vi "Mem_Release.vi"(8 "error in (no error)":errorcluster, 11 "AddrQueueIn":refnum<queue>) -> (0 "error out":errorcluster)   [LabVIEW 2019, in "Memory Data Access.lvlib"]
uses:
  Memory Data Access.lvlib
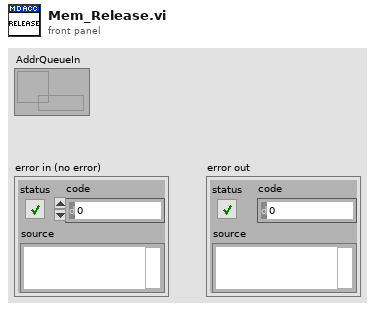
[diagram p1: front panel]
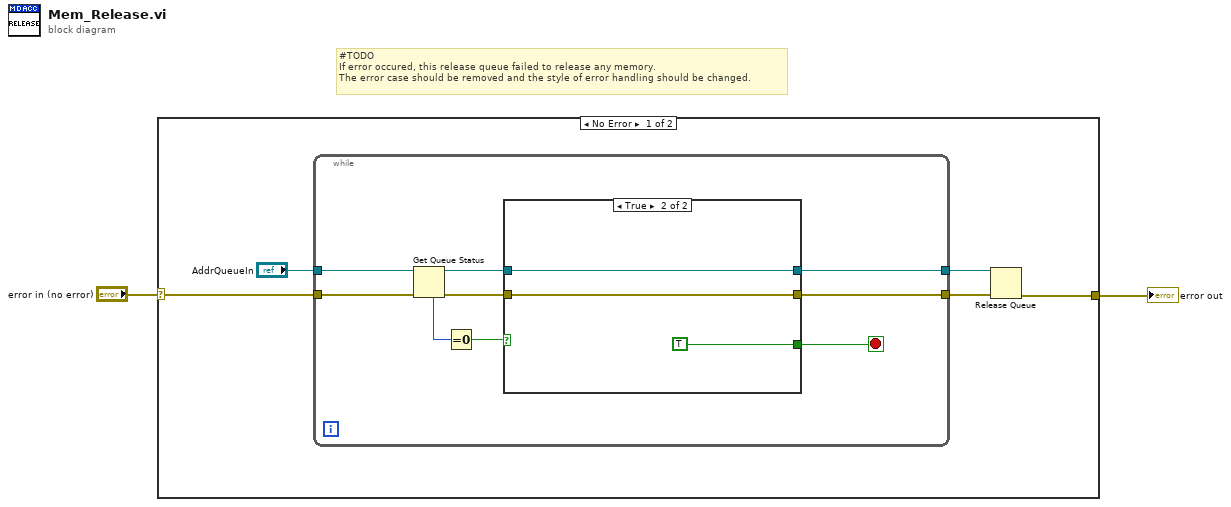
[diagram p0: block diagram]
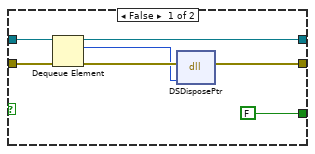
[diagram p2: hidden frame]
diagram:
  # "#TODO\nIf error occured, this release queue failed to release any memory.\nThe error case should be removed and the style of error handling should be changed."
  n1 = case shown="No Error" "error in (no error)" {
    selector: "error in (no error)" -> [w6 w27]
    tunnel: [w3 w27] -> w1
    frame No Error {
      n2 = while {
        tunnel: "AddrQueueIn" -> [w16]
        tunnel: [w10] -> w5
        tunnel: [w9] -> w4
        tunnel: w6 -> [w8]
        stop <- w13 stop-if-true
        n3 = Get Queue Status(queue=w16, error in (no error)=w8) -> (queue out=w12:refnum<queue>, error out=w11:errorcluster, # elements in queue=w15:i32)  [unwired: 1 in, 5 out]
        n4 = Equal To 0?(x=w15) -> (x = 0?=w14:bool)
        n5 = case shown="True" w14 {
          tunnel: [FALSE TRUE] -> w13
          tunnel: w12 -> [w23 w25]
          tunnel: w11 -> [w22 w24]
          tunnel: [w21 w25] -> w10
          tunnel: [w18 w24] -> w9
          frame False {
            n6 = Dequeue Element(queue=w23, error in (no error)=w22) -> (queue out=w21:refnum<queue>, element=w19:u64, error out=w20:errorcluster)  [unwired: 1 in, 1 out]
            n7 = dll-call lib="LabVIEW" fn="DSDisposePtr"(error in=w20, "Pointer"=w19) -> (error out=w18:errorcluster)  [unwired: 4 in, 1 out]
          }
          frame True {
          }
        }
      }
      n8 = Release Queue(queue=w5, error in (no error)=w4) -> (error out=w3:errorcluster)  [unwired: 1 in, 2 out]
    }
    frame Error {
    }
  }
  "error out" <- w1
